vi "Dispatch Group.vi"(7 "command":T1, 8 "error in (no error)":errorcluster, 9 "Plugin ID":i32, 10 "Dispatcher Interface in":refnum<class "Dispatcher Interface.lvclass">, 11 "Scheduler Transfer Group Bundle in":refnum<class "Scheduler Transfer Group Bundle.lvclass">) -> (0 "error out":errorcluster, 2 "Dispatcher Interface out":refnum<class "Dispatcher Interface.lvclass">, 3 "Scheduler Transfer Group Bundle out":refnum<class "Scheduler Transfer Group Bundle.lvclass">)   [LabVIEW 2017, in "DSF Core.lvlib" / "Scheduler Transfer Group Bundle.lvclass"]
uses:
  Scheduler Transfer Group Bundle.lvclass
  Interfaces/Dispatcher/Dispatcher Interface.lvclass
  Interfaces/Dispatcher/Command.ctl
  Scheduler Transfer Group Bundle.lvclass/Scheduler Transfer Group Bundle.ctl
  Timing/Timing.lvclass/Timing.ctl
  Timing/Transfer Group Timing.lvclass
  C:/Git/DSF/Data Sharing Framework/Source/Core/Engine/Classes/Timing/Timing.lvclass
  Timing/Timing.lvclass
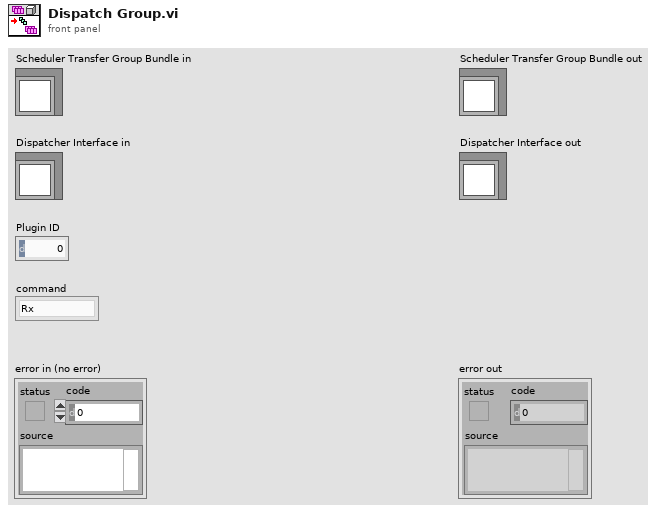
[diagram p1: front panel]
types:
  T1 = typedef "DSF Core.lvlib/Dispatcher Interface.lvclass/Command.ctl" = enum8{"Rx", "Tx", "Shutdown"}
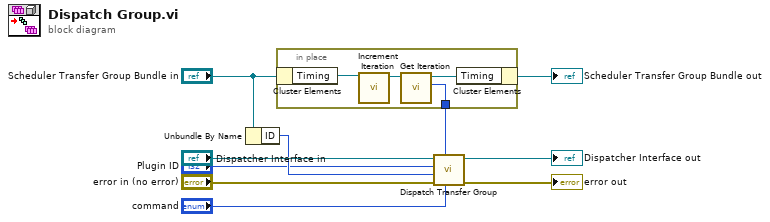
[diagram p0: block diagram]
diagram:
  n1 = Unbundle By Name("Scheduler Transfer Group Bundle in") -> ("ID"=w8:i32)
  n2 = in-place {
    in-place-border: [w11] -> w6
    n3 = in-place-cluster #1("Scheduler Transfer Group Bundle in") -> ("Timing"=w14:refnum<class "Transfer Group Timing.lvclass">)
    n4 = call "Increment Iteration.vi"("Timing in"=w14) -> ("Timing out"=w13:refnum<class "Transfer Group Timing.lvclass">)  [unwired: 10 in]
    n5 = call "Get Iteration.vi"("Timing in"=w13) -> ("Iteration"=w11:u64, "Timing out"=w12:refnum<class "Transfer Group Timing.lvclass">)  [unwired: 9 in]
    n6 = in-place-cluster #1("Timing"=w12) -> (→"Scheduler Transfer Group Bundle out":refnum<class "Scheduler Transfer Group Bundle.lvclass">)
  }
  n7 = call "Dispatch Transfer Group.vi"("command"="command", "Iteration"=w6, "error in (no error)"="error in (no error)", "Transfer Group ID"=w8, "Plugin ID"="Plugin ID", "Dispatcher Interface in"="Dispatcher Interface in") -> ("error out"=→"error out":errorcluster, "Dispatcher Interface out"=→"Dispatcher Interface out":refnum<class "Dispatcher Interface.lvclass">)  [unwired: 4 in]
